vi "Draw Bar Line.vi"(9 "Line Length":i16, 10 "end point":cluster{"x":i16, "y":i16}, 11 "picture in":picture) -> (3 "picture out":picture)   [LabVIEW 2014]
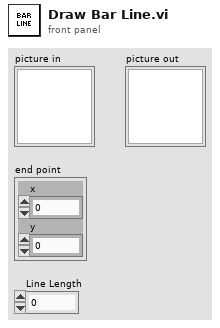
[diagram p1: front panel]
types:
  T1 = cluster{"Width":u16, "Style":enum32{"Solid", "Dash", "Dot", "DashDot", "DashDotDot"}}
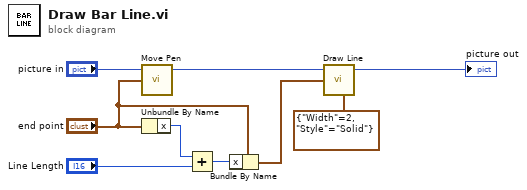
[diagram p0: block diagram]
diagram:
  n1 = call <vilib>:"Move Pen.vi"("new position"="end point", "picture"="picture in") -> ("new picture"=w8:picture)  [unwired: 3 in]
  n2 = Unbundle By Name("end point") -> ("x"=w3:i16)
  n3 = Add(x=w3, y="Line Length") -> (x+y=w5:i16)
  n4 = Bundle By Name(cluster="end point", "x"=w5) -> (w2:cluster{"x":i16, "y":i16})
  n5 = call <vilib>:"Draw Line.vi"("picture"=w8, "end point"=w2, "pen"=T1 {"Width"=2, "Style"=enum."Solid"}) -> ("new picture"=→"picture out":picture)  [unwired: 6 in]
